vi "Open.vi"(8 "error in (no error)":errorcluster, 10 "Update Rate (4Hz-100Hz)":u8=100, 11 "navX - Base in":refnum<class "navX - Base.lvclass">) -> (0 "error out":errorcluster, 3 "navX - Base out":refnum<class "navX - Base.lvclass">)   [LabVIEW 2015, in "navX Library v3.lvlib" / "navX - Base.lvclass"]
uses:
  navX - Base.lvclass
  navX Registry Cache/navX Registry Cache.lvclass
  navX - Base.lvclass/navX - Base.ctl
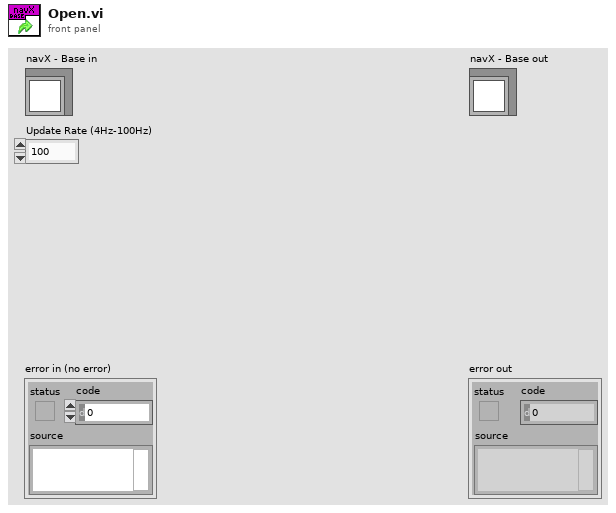
[diagram p1: front panel]
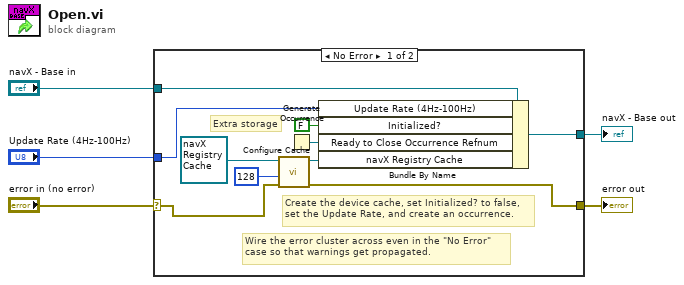
[diagram p0: block diagram]
diagram:
  n1 = case shown="No Error" "error in (no error)" {
    selector: "error in (no error)" -> [w7 w17]
    tunnel: [w8 w17] -> w4
    tunnel: [w9 w16] -> w2
    tunnel: "navX - Base in" -> [w10 w16]
    tunnel: "Update Rate (4Hz-100Hz)" -> [w6 _]
    frame No Error {
      # "Extra storage"
      # "Create the device cache, set Initialized? to false,\nset the Update Rate, and create an occurrence."
      # "Wire the error cluster across even in the \"No Error\"\ncase so that warnings get propagated."
      n2 = call "Configure Cache.vi"("error in (no error)"=w7, "Cache Size"=128 ("dimension size"), "navX Registry Cache in"=refnum<class "navX Registry Cache.lvclass"> refnum ("navX Library v3.lvlib:navX Registry Cache.lvclass")) -> ("error out"=w8:errorcluster, "navX Registry Cache out"=w13:refnum<class "navX Registry Cache.lvclass">)  [unwired: 7 in]
      n3 = Generate Occurrence() -> (w15:refnum<k4>)
      n4 = Bundle By Name(cluster=w10, "Update Rate (4Hz-100Hz)"=w6, "Initialized?"=FALSE, "Ready to Close Occurrence Refnum"=w15, "navX Registry Cache"=w13) -> (w9:refnum<class "navX - Base.lvclass">)
    }
    frame Error {
    }
  }
  "error out" <- w4
  "navX - Base out" <- w2
